vi "TargetExperimentalSetup_flux.vi"() -> ()   [LabVIEW 2015]
uses:
  <vilib>/userdefined/High Color/IMAQdx.ctl
  <vilib>/DAQmx/read.llb/DAQmx Read (Analog 1D DBL NChan 1Samp).vi
  <vilib>/DAQmx/read.llb/DAQmx Read (Analog DBL 1Chan 1Samp).vi
  <vilib>/DAQmx/miscellaneous.llb/DAQmx Fill In Error Info.vi
  <vilib>/Utility/file.llb/Write Delimited Spreadsheet (string).vi
  <instrlib>/Zaber A Series/Zaber A Series.lvlib
  <vilib>/vision/driver/NI_Vision_Acquisition_Software.lvlib
  <resource>/objmgr/imaqdx.rc
panel:
  in  "Y Coordinate":i32=50
  in  "X Coordinate":i32=50
  in  "Diameter":i32=10
  out "Image 2":T1(plugin-control)
  in  "Capture":bool
  out "Monochromatic Camera":errorcluster
  in  "Exposure Time (µs)":dbl=900000.0
  in  "Gamma Enabled":bool=TRUE
  in  "Frame Rate (hz)":dbl=24.0
  in  "Black Level":dbl(slide) scale=0.0..100.0
  out "Observer Camera":errorcluster
  in  "Exposure Time (µs)":dbl=100000.0
  in  "Gamma Enabled 2":bool=TRUE
  in  "Frame Rate (hz)":dbl=15.0
  in  "Black Level":dbl(slide) scale=0.0..100.0
  out "Flowmeter":errorcluster
  out "Thermocouple":errorcluster
  out "Actuator":errorcluster
  in  "Record":bool
  in  "Fluxmeter Data File":path
  in  "Image Folder Path":path
  out "Heat Flux (W/cm2)":string
  out "Fluxmeter":dbl(knob) scale=0.0..1200.0
  out "High Flux \nWarning":bool
  out "High Temp Warning":bool
  in  "Set Speed":bool
  out "Image":T1(plugin-control)
  in  "Step Increment (+/-)":string="10"
  out "Mass Flow (g/s)":string
  out "Mass Flow Inlet":dbl(knob) scale=0.0..150.0
  in  "Record Time (s)":u16=1 min=1
  in  "Lamp Number":dbl
  out "Filename":string
  in  "OK Button 2":bool
  out "Water Outlet - Fluxmeter":dbl(knob) scale=0.0..100.0
  out "Water Outlet - Target":dbl(knob) scale=0.0..100.0
  out "Water Inlet - Fluxmeter":dbl(knob) scale=0.0..100.0
  in  "?":bool
  out "High Temp Warning":bool
  out "High Temp \nWarning":bool
  out "Temperature (C°)":string
  out "Temperature (C°)":string
  out "Temperature (C°)":string
  out "End Reached":bool
  in  "?":bool
  out "Actuator Status":bool
  out "Position":string
  in  "?":bool
  in  "Speed (%)":string="35"
  in  "Set Position \n(150 <-> -150)":string="0"
  # "LINEAR ACTUATOR CONTROL"
  # "CAMERA FEEDS"
  # "CAMERA CONTROL"
  # "Monochromatic Camera"
  # "Observer Camera"
  # "HEAT FLUXMETER DISPLAY"
  # "HARDWARE CHECKLIST"
  # "NI 9211 THERMOCOUPLE MODULE DISPLAY"
  # "NI 9207 VOLTAGE AND CURRENT MODULE"
  # "Finding label on image"
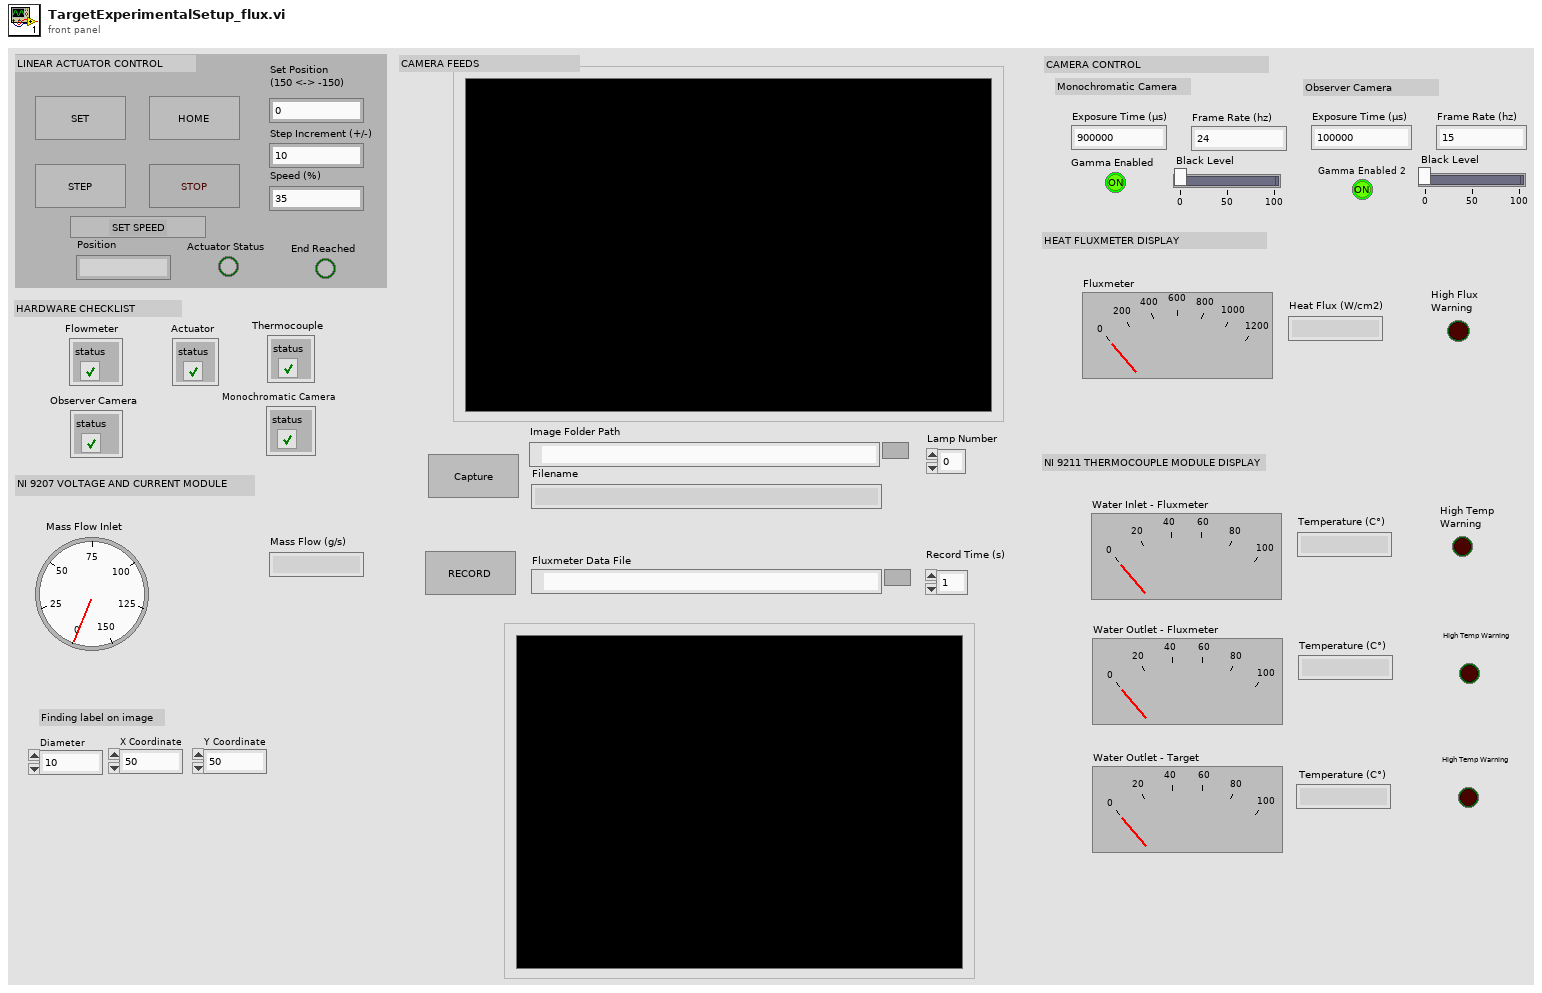
[diagram p1: front panel]
types:
  T1 = typedef "IMAQ Image.ctl" = refnum<image>
  T2 = cluster{"Left":i32, "Top":i32, "Right":i32, "Bottom":i32}
  T3 = typedef "IMAQdx.ctl" = refnum<k21>
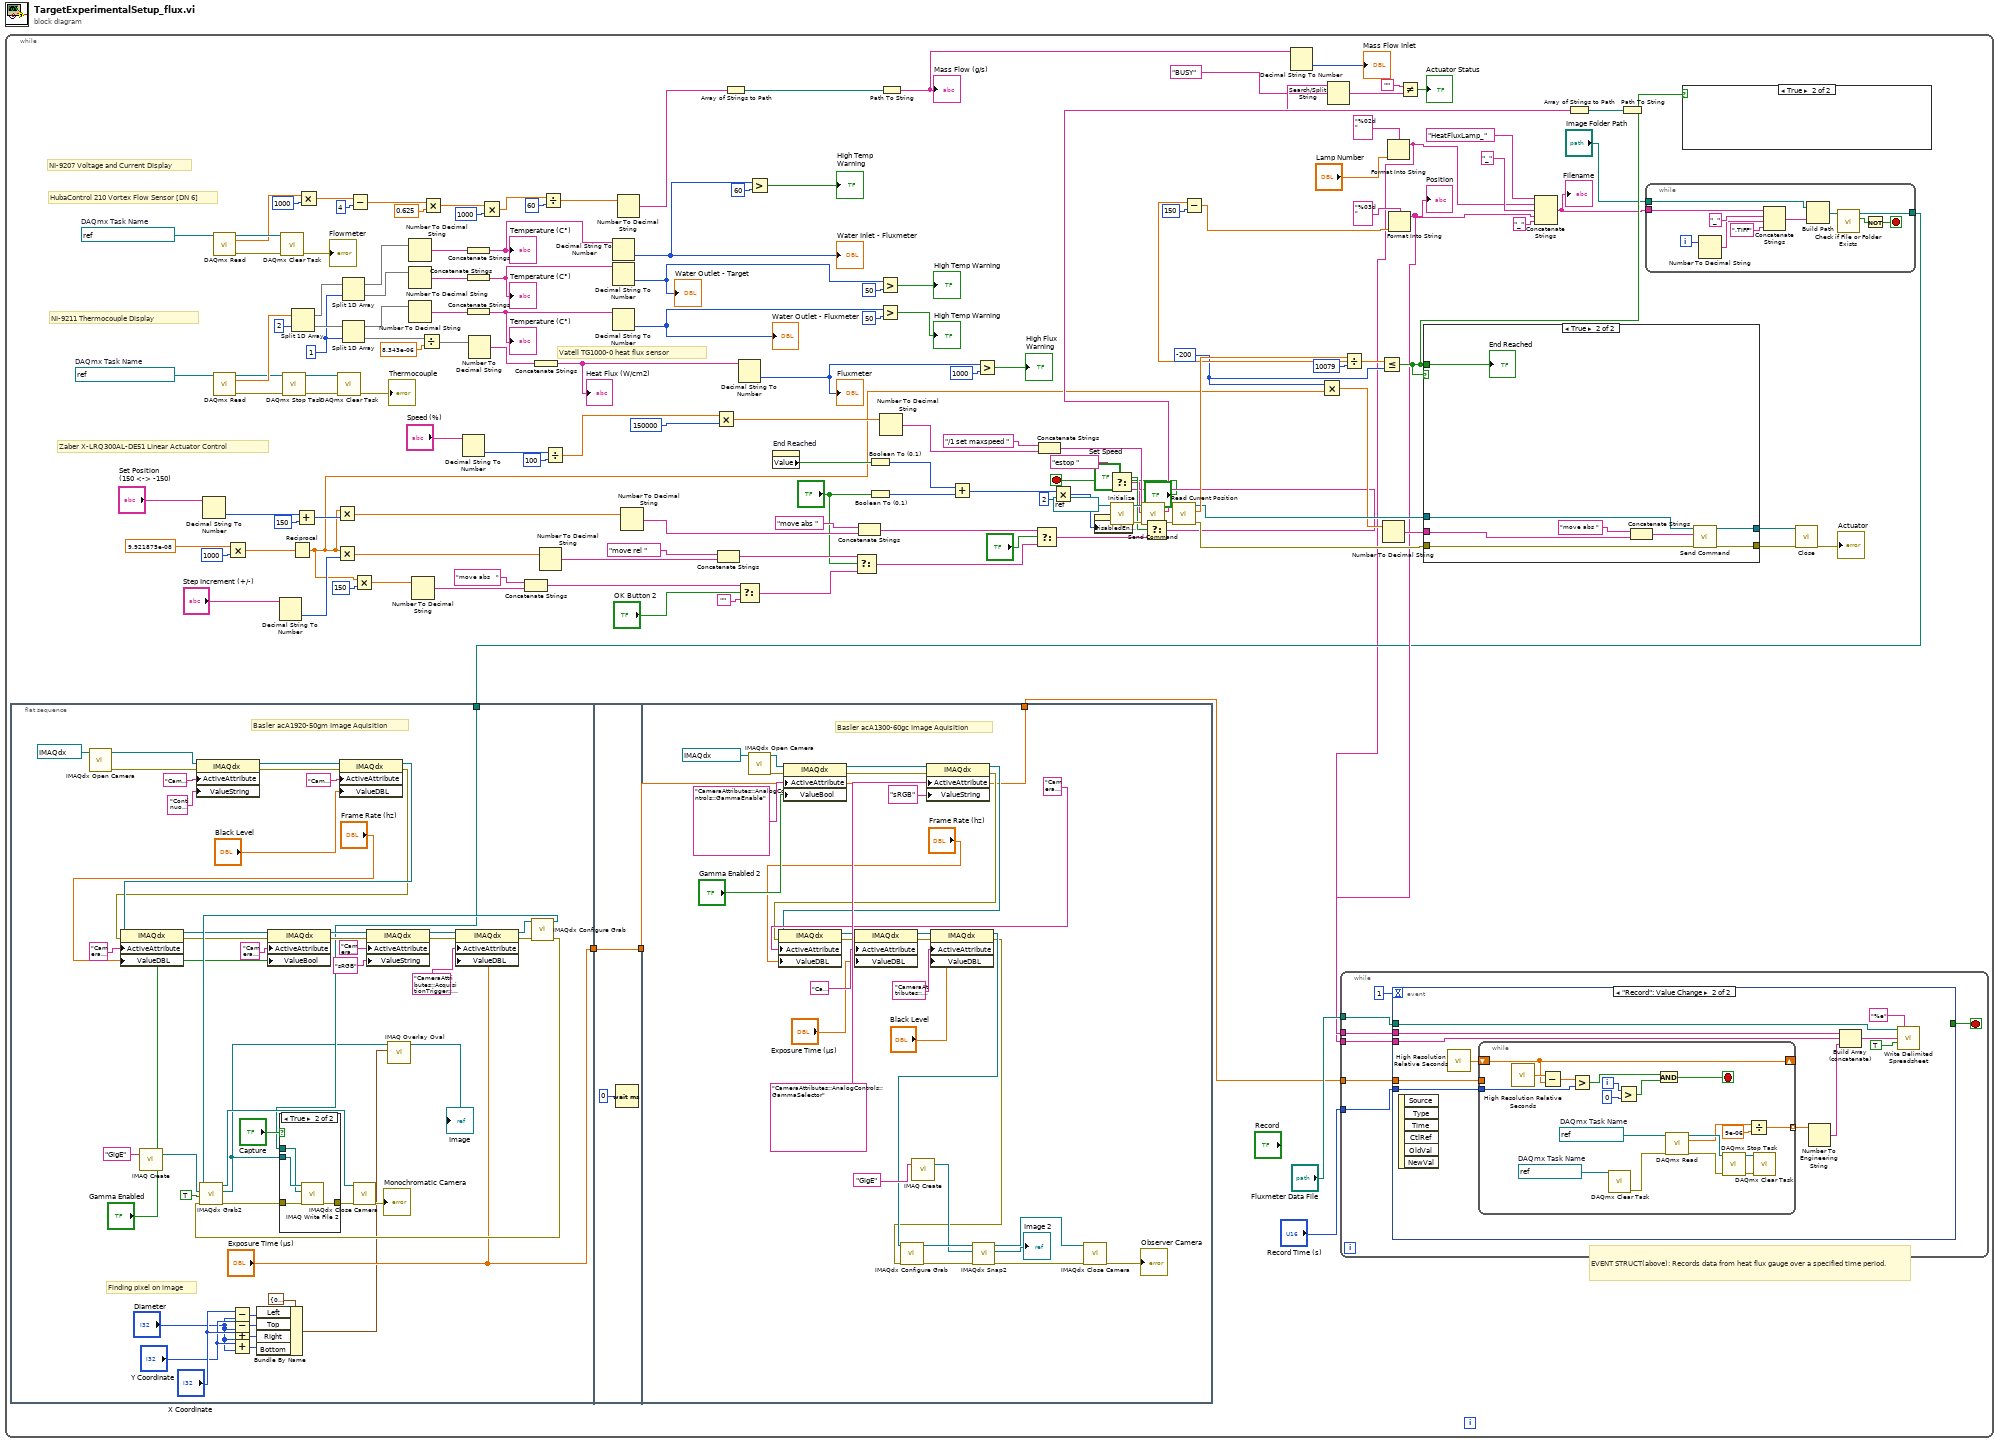
[diagram p0: block diagram]
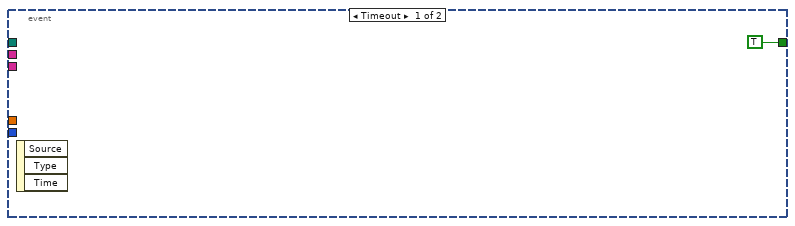
[diagram p3: hidden frame]
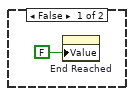
[diagram p4: hidden frame]
diagram:
  n1 = while {
    stop <- "?" stop-if-true
    w43 = refnum<k21> "Flowmeter-Current"  # DAQmx Task Name
    w103 = 1
    w35 = refnum<k21> "MyTemperatureTask"  # DAQmx Task Name
    w62 = -200
    # "Vatell TG1000-0 heat flux sensor"
    # "Zaber X-LRQ300AL-DE51 Linear Actuator Control"
    # "EVENT STRUCT(above): Records data from heat flux gauge over a specified time period."
    # "HubaControl 210 Vortex Flow Sensor [DN 6]"
    # "NI-9207 Voltage and Current Display"
    # "NI-9211 Thermocouple Display"
    n2 = flat-sequence {
      tunnel: ["Exposure Time (µs)"] -> w2
      tunnel: w4 -> [w161]
      tunnel: w2 -> [w202]
      tunnel: [w202] -> w1
      tunnel: [w204] -> w5
      tunnel: w1 -> [w204]
      frame #0 {
        # "Finding pixel on image"
        # "Basler acA1920-50gm Image Aquisition"
        n3 = call <vilib>:"IMAQdx Open Camera.vi"("Session In"=T3 "Mono" ("IMAQdx Session")) -> ("error out"=w169:errorcluster, "Session Out"=w170:T3)  [unwired: 9 in]
        n4 = call "IMAQ Create"("Image Name"="GigE") -> ("New Image"=w196:T1)  [unwired: 4 in, 1 out]
        n5 = property class="IMAQdx"(reference=w170, error in=w169, "ActiveAttribute"="CameraAttributes::AnalogControls::GainAuto", "ValueString"="Continuous") -> (reference out=w176:T3, error out=w174:errorcluster)
        n6 = Subtract(x="X Coordinate", y="Diameter") -> (x-y=w158:i32)
        n7 = Subtract(x="Y Coordinate", y="Diameter") -> (x-y=w155:i32)
        n8 = Add(x="X Coordinate", y="Diameter") -> (x+y=w156:i32)
        n9 = Add(x="Y Coordinate", y="Diameter") -> (x+y=w157:i32)
        n10 = Bundle By Name(cluster=T2 {"Left"=0, "Top"=0, "Right"=0, "Bottom"=0} ("Bounding Rectangle"), "Left"=w158, "Top"=w155, "Right"=w156, "Bottom"=w157) -> (w151:T2)
        n11 = property class="IMAQdx"(reference=w176, error in=w174, "ActiveAttribute"="CameraAttributes::AnalogControls::BlackLevelRaw", "ValueDBL"="Black Level") -> (reference out=w175:T3, error out=w173:errorcluster)
        n12 = property class="IMAQdx"(reference=w175, error in=w173, "ActiveAttribute"="CameraAttributes::AcquisitionTrigger::AcquisitionFrameRateAbs", "ValueDBL"="Frame Rate (hz)") -> (reference out=w179:T3, error out=w178:errorcluster)
        n13 = property class="IMAQdx"(reference=w179, error in=w178, "ActiveAttribute"="CameraAttributes::AnalogControls::GammaEnable", "ValueBool"="Gamma Enabled") -> (reference out=w191:T3, error out=w185:errorcluster)
        n14 = property class="IMAQdx"(reference=w191, error in=w185, "ActiveAttribute"="CameraAttributes::AnalogControls::GammaSelector", "ValueString"="sRGB") -> (reference out=w190:T3, error out=w184:errorcluster)
        n15 = property class="IMAQdx"(reference=w190, error in=w184, "ActiveAttribute"="CameraAttributes::AcquisitionTrigger::ExposureTimeAbs", "ValueDBL"="Exposure Time (µs)") -> (reference out=w188:T3, error out=w183:errorcluster)
        n16 = call <vilib>:"IMAQdx Configure Grab.vi"("error in"=w183, "Session In"=w188) -> ("error out"=w182:errorcluster, "Session Out"=w194:T3)  [unwired: 8 in]
        n17 = call <vilib>:"IMAQdx Grab2.vi"("error in"=w182, "Wait for Next Buffer? (Yes)"=TRUE, "Image In"=w196, "Session In"=w194) -> ("error out"=w163:errorcluster, "Image Out"=w150:T1, "Session Out"=w193:T3)  [unwired: 4 in, 1 out]
        n18 = case shown="True" "Capture" {
          tunnel: w150 -> [_ w199]
          tunnel: w163 -> [_ w201]
          tunnel: [_ w200] -> w162
          tunnel: w161 -> [_ w198]
          frame False {
          }
          frame True {
            n19 = call-poly "IMAQ Write File 2"("error in (no error)"=w201, "File Path"=w198, "Image"=w199) -> ("error out"=w200:errorcluster)  [unwired: 7 in, 1 out]
          }
        }
        n20 = call <vilib>:"IMAQdx Close Camera.vi"("error in"=w162, "Session In"=w193) -> ("error out"=→"Monochromatic Camera":errorcluster)  [unwired: 9 in]
        n21 = call "IMAQ Overlay Oval"("Bounding Rectangle"=w151, "Image"=w150) -> ("Image Out"=→"Image":T1)  [unwired: 8 in, 1 out]
      }
      frame #1 {
        n22 = Wait (ms)(milliseconds to wait=0) -> ()  [unwired: 1 out]
      }
      frame #2 {
        # "Basler acA1300-60gc Image Aquisition"
        n23 = call <vilib>:"IMAQdx Open Camera.vi"("Session In"=T3 "GIE1300-1" ("IMAQdx Session 2")) -> ("error out"=w215:errorcluster, "Session Out"=w216:T3)  [unwired: 9 in]
        n24 = property class="IMAQdx"(reference=w216, error in=w215, "ActiveAttribute"="CameraAttributes::AnalogControls::GammaEnable", "ValueBool"="Gamma Enabled 2") -> (reference out=w234:T3, error out=w231:errorcluster)
        n25 = call "IMAQ Create"("Image Name"="GigE") -> ("New Image"=w226:T1)  [unwired: 4 in, 1 out]
        n26 = property class="IMAQdx"(reference=w234, error in=w231, "ActiveAttribute"="CameraAttributes::AnalogControls::GammaSelector", "ValueString"="sRGB") -> (reference out=w221:T3, error out=w220:errorcluster)
        n27 = property class="IMAQdx"(reference=w221, error in=w220, "ActiveAttribute"="CameraAttributes::AcquisitionTrigger::AcquisitionFrameRateAbs", "ValueDBL"="Frame Rate (hz)") -> (reference out=w218:T3, error out=w217:errorcluster)
        n28 = property class="IMAQdx"(reference=w218, error in=w217, "ActiveAttribute"="CameraAttributes::AcquisitionTrigger::ExposureTimeAbs", "ValueDBL"="Exposure Time (µs)") -> (reference out=w212:T3, error out=w211:errorcluster)
        n29 = property class="IMAQdx"(reference=w212, error in=w211, "ActiveAttribute"="CameraAttributes::AnalogControls::BlackLevelRaw", "ValueDBL"="Black Level") -> (reference out=w208:T3, error out=w207:errorcluster)
        n30 = call <vilib>:"IMAQdx Configure Grab.vi"("error in"=w207, "Session In"=w208) -> ("error out"=w229:errorcluster, "Session Out"=w228:T3)  [unwired: 8 in]
        n31 = call <vilib>:"IMAQdx Snap2.vi"("error in"=w229, "Image In"=w226, "Session In"=w228) -> ("error out"=w223:errorcluster, "Image Out"=→"Image 2":T1, "Session Out"=w225:T3)  [unwired: 6 in]
        n32 = call <vilib>:"IMAQdx Close Camera.vi"("error in"=w223, "Session In"=w225) -> ("error out"=→"Observer Camera":errorcluster)  [unwired: 9 in]
      }
    }
    n33 = Decimal String To Number(string="Set Position \n(150 <-> -150)") -> (number=w91:i32)  [unwired: 2 in, 1 out]
    n34 = call-poly <vilib>:"DAQmx Read.vi"("task/channels in"=w43) -> ("task out"=w45:refnum<k21>, "data"=w34:dbl[], "error out"=w44:errorcluster)  [unwired: 12 in]
    n35 = call-poly <vilib>:"DAQmx Read.vi"("task/channels in"=w35) -> ("task out"=w16:refnum<k21>, "data"=w107:dbl[], "error out"=w15:errorcluster)  [unwired: 12 in]
    n36 = Multiply(x=9.921875e-08, y=1000) -> (x*y=w145:dbl)
    n37 = Decimal String To Number(string="Step Increment (+/-)") -> (number=w89:i32)  [unwired: 2 in, 1 out]
    n38 = call <vilib>:"DAQmx Clear Task.vi"("task in"=w45, "error in"=w44) -> ("error out"=→"Flowmeter":errorcluster)  [unwired: 13 in]
    n39 = call <vilib>:"DAQmx Stop Task.vi"("task/channels in"=w16, "error in"=w15) -> ("task out"=w14:refnum<k21>, "error out"=w13:errorcluster)  [unwired: 12 in]
    n40 = Reciprocal(x=w145) -> (1/x=w70:dbl)
    n41 = Split 1D Array(array=w107, index=2) -> (first subarray=w105:dbl[], second subarray=w104:dbl[])
    n42 = Add(x=w91, y=150) -> (x+y=w94:i32)
    n43 = Multiply(x=w34, y=1000) -> (x*y=w32:dbl[])
    n44 = Multiply(x=w70, y=w94) -> (x*y=w93:dbl)
    n45 = Multiply(x=w70, y=w89) -> (x*y=w130:dbl)
    n46 = call <vilib>:"DAQmx Clear Task.vi"("task in"=w14, "error in"=w13) -> ("error out"=→"Thermocouple":errorcluster)  [unwired: 13 in]
    n47 = Split 1D Array(array=w105, index=w103) -> (first subarray=w100:dbl[], second subarray=w102:dbl[])
    n48 = Split 1D Array(array=w104, index=w103) -> (first subarray=w101:dbl[], second subarray=w38:dbl[])
    n49 = Subtract(x=w32, y=4) -> (x-y=w48:dbl[])
    n50 = Multiply(x=w70, y=150) -> (x*y=w72:dbl)
    n51 = Number To Decimal String(number=w100) -> (decimal integer string=w26:string[])  [unwired: 1 in]
    n52 = Number To Decimal String(number=w102) -> (decimal integer string=w28:string[])  [unwired: 1 in]
    n53 = Number To Decimal String(number=w101) -> (decimal integer string=w30:string[])  [unwired: 1 in]
    n54 = Number To Decimal String(number=w72) -> (decimal integer string=w75:string)  [unwired: 1 in]
    n55 = Divide(x=w38, y=8.343e-06) -> (x/y=w17:dbl[])
    n56 = Multiply(x=w48, y=0.625) -> (x*y=w57:dbl[])
    n57 = Decimal String To Number(string="Speed (%)") -> (number=w82:i32)  [unwired: 2 in, 1 out]
    n58 = Concatenate Strings(w26) -> (w25:string)
    "Temperature (C°)" <- w25
    n59 = Concatenate Strings(w28) -> (w27:string)
    "Temperature (C°)" <- w27
    n60 = Concatenate Strings(w30) -> (w29:string)
    "Temperature (C°)" <- w29
    n61 = Number To Decimal String(number=w17) -> (decimal integer string=w31:string[])  [unwired: 1 in]
    n62 = Multiply(x=w57, y=1000) -> (x*y=w55:dbl[])
    n63 = Concatenate Strings("move abs   ", w75) -> (w71:string)
    n64 = Concatenate Strings(w31) -> (w7:string)
    "Heat Flux (W/cm2)" <- w7
    n65 = Number To Decimal String(number=w130) -> (decimal integer string=w128:string)  [unwired: 1 in]
    n66 = Divide(x=w55, y=60) -> (x/y=w58:dbl[])
    n67 = Divide(x=w82, y=100) -> (x/y=w79:dbl)
    n68 = Decimal String To Number(string=w25) -> (number=w61:i32)  [unwired: 2 in, 1 out]
    "Water Inlet - Fluxmeter" <- w61
    n69 = Decimal String To Number(string=w27) -> (number=w24:i32)  [unwired: 2 in, 1 out]
    "Water Outlet - Target" <- w24
    n70 = Decimal String To Number(string=w29) -> (number=w20:i32)  [unwired: 2 in, 1 out]
    "Water Outlet - Fluxmeter" <- w20
    n71 = Number To Decimal String(number=w58) -> (decimal integer string=w50:string[])  [unwired: 1 in]
    n72 = Number To Decimal String(number=w93) -> (decimal integer string=w143:string)  [unwired: 1 in]
    n73 = Multiply(x=w79, y=150000) -> (x*y=w78:dbl)
    n74 = Concatenate Strings("move rel ", w128) -> (w127:string)
    n75 = Array of Strings to Path(0:w50) -> (2:w51:path)  [unwired: 1 in]
    n76 = Decimal String To Number(string=w7) -> (number=w41:i32)  [unwired: 2 in, 1 out]
    "Fluxmeter" <- w41
    n77 = Select(t=w71, s="OK Button 2", f="") -> (s? t:f=w69:string)
    n78 = Greater?(x=w61, y=60) -> (0:→"High Temp \nWarning":bool)
    n79 = property on="End Reached" class="Bool (strict)"() -> ("Value"=w120:bool)  [unwired: 2 in, 2 out]
    n80 = Select(t=w127, s="?", f=w69) -> (s? t:f=w126:string)
    n81 = Concatenate Strings("move abs ", w143) -> (w125:string)
    n82 = Boolean To (0,1)(Boolean=w120) -> (0, 1=w119:i16)
    n83 = Boolean To (0,1)(Boolean="?") -> (0, 1=w121:i16)
    n84 = Greater?(x=w24, y=50) -> (0:→"High Temp Warning":bool)
    n85 = Greater?(x=w20, y=50) -> (0:→"High Temp Warning":bool)
    n86 = Number To Decimal String(number=w78) -> (decimal integer string=w86:string)  [unwired: 1 in]
    n87 = Path To String(path=w51) -> (string=w53:string)
    "Mass Flow (g/s)" <- w53
    n88 = Add(x=w119, y=w121) -> (x+y=w118:i16)
    n89 = Greater?(x=w41, y=1000) -> (0:→"High Flux \nWarning":bool)
    n90 = Select(t=w125, s="?", f=w126) -> (s? t:f=w83:string)
    n91 = Concatenate Strings("/1 set maxspeed ", w86) -> (w84:string)
    n92 = Multiply(x=w118, y=2) -> (x*y=w114:i32)
    n93 = property class="Bool"("DisabledEnum"=w114) -> ()  [unwired: 2 in, 2 out]
    n94 = call <instrlib>:"Initialize.vi"("VISA resource name"=refnum<visa-resource-name> "COM3") -> ("error out"=w113:errorcluster, "VISA resource name out"=w141:refnum<visa-resource-name>)  [unwired: 9 in]
    n95 = Select(t=w84, s="Set Speed", f=w83) -> (s? t:f=w67:string)
    n96 = Select(t="estop ", s="?", f=w67) -> (s? t:f=w66:string)
    n97 = call <instrlib>:"Send Command.vi"("error in (no error)"=w113, "Command"=w66, "VISA resource name"=w141) -> ("error out"=w112:errorcluster, "Response String Array"=w136:string[], "VISA resource name out"=w140:refnum<visa-resource-name>)  [unwired: 4 in, 2 out]
    n98 = call <instrlib>:"Read Current Position.vi"("error in (no error)"=w112, "VISA resource name"=w140) -> ("error out"=w111:errorcluster, "Position"=w139:dbl, "VISA resource name out"=w117:refnum<visa-resource-name>)  [unwired: 7 in]
    n99 = Decimal String To Number(string=w53) -> (number=→"Mass Flow Inlet":i32)  [unwired: 2 in, 1 out]
    n100 = Multiply(x=w62, y=w70) -> (x*y=w116:dbl)
    n101 = Divide(x=w139, y=10079) -> (x/y=w63:dbl)
    n102 = Subtract(x=w63, y=150) -> (x-y=w18:dbl)
    n103 = Less Or Equal?(x=w63, y=w62) -> (x <= y?=w64:bool)
    n104 = Number To Decimal String(number=w116) -> (decimal integer string=w115:string)  [unwired: 1 in]
    n105 = Format Into String(format string="%02d", "Lamp Number") -> (resulting string=w3:string)  [unwired: 2 in, 1 out]
    n106 = Format Into String(format string="%03d", w18) -> (resulting string=w9:string)  [unwired: 2 in, 1 out]
    "Position" <- w9
    n107 = while {
      tunnel: "Fluxmeter Data File" -> [w240]
      tunnel: w3 -> [w239]
      tunnel: w9 -> [w238]
      tunnel: w5 -> [w237]
      tunnel: "Record Time (s)" -> [w236]
      stop <- w241 stop-if-true
      n108 = event shown="[1] \"Record\": Value Change" {
        selector: _ -> [_ _]
        dyn-events: _ -> [_ _]
        timeout: 1 -> [_ _]
        tunnel: [TRUE _] -> w241
        tunnel: w240 -> [_ w254]
        tunnel: w239 -> [_ w250]
        tunnel: w238 -> [_ w249]
        tunnel: w237 -> [_ w247]
        tunnel: w236 -> [_ w244]
        event Timeout {
          n109 = event-data() -> ()  [unwired: 1 in, 3 out]
        }
        event "Record": Value Change {
          n110 = event-data() -> ()  [unwired: 1 in, 6 out]
          n111 = call <vilib>:"High Resolution Relative Seconds.vi"() -> ("relative seconds"=w246:dbl)
          n112 = while {
            tunnel: [w257] -> w252 mode=indexing
            shift-right: [w259] -> _
            shift-left: w246 -> [w259]
            tunnel: w247 -> [_]
            tunnel: w244 -> [w255]
            i -> [w266]
            stop <- w261 stop-if-true
            w268 = refnum<k21> "HF-Voltage"  # DAQmx Task Name
            w273 = refnum<k21> "HF-Voltage"  # DAQmx Task Name
            n113 = call <vilib>:"High Resolution Relative Seconds.vi"() -> ("relative seconds"=w260:dbl)
            n114 = Subtract(x=w260, y=w259) -> (x-y=w264:dbl)
            n115 = Greater?(x=w264, y=w255) -> (0:w263:bool)
            n116 = call <vilib>:"DAQmx Clear Task.vi"("task in"=w268) -> ("error out"=w267:errorcluster)  [unwired: 14 in]
            n117 = Greater?(x=w266, y=0) -> (0:w262:bool)
            n118 = And(x=w263, y=w262) -> (x .and. y?=w261:bool)
            n119 = call-poly <vilib>:"DAQmx Read.vi"("task/channels in"=w273, "error in"=w267) -> ("task out"=w272:refnum<k21>, "data"=w256:dbl, "error out"=w271:errorcluster)  [unwired: 11 in]
            n120 = call <vilib>:"DAQmx Stop Task.vi"("task/channels in"=w272, "error in"=w271) -> ("task out"=w270:refnum<k21>, "error out"=w269:errorcluster)  [unwired: 12 in]
            n121 = Divide(x=w256, y=9e-06) -> (x/y=w257:dbl)
            n122 = call <vilib>:"DAQmx Clear Task.vi"("task in"=w270, "error in"=w269) -> ()  [unwired: 13 in, 1 out]
          }
          n123 = Number To Engineering String(4:w252) -> (0:w251:string[])  [unwired: 3 in]
          n124 = Build Array (concatenate)(w249, w250, w251) -> (w248:string[])
          n125 = call-poly <vilib>:"Write Delimited Spreadsheet.vi"("file path (dialog if empty)"=w254, "format (%s)"="%e", "1D data"=w248, "append to file? (F)"=TRUE) -> ()  [unwired: 10 in, 2 out]
        }
      }
    }
    n126 = case shown="True" w64 {
      tunnel: w64 -> [_ w293]
      tunnel: w117 -> [_ w292]
      tunnel: w115 -> [_ w289]
      tunnel: w111 -> [_ w288]
      tunnel: [_ w287] -> w110
      tunnel: [_ w286] -> w108
      frame False {
      }
      frame True {
        n127 = Concatenate Strings("move abs ", w289) -> (w290:string)
        n128 = call <instrlib>:"Send Command.vi"("error in (no error)"=w288, "Command"=w290, "VISA resource name"=w292) -> ("error out"=w287:errorcluster, "VISA resource name out"=w286:refnum<visa-resource-name>)  [unwired: 4 in, 3 out]
        "End Reached" <- w293
      }
    }
    n129 = Concatenate Strings("HeatFluxLamp_", w3, "_", w9, "_") -> (w36:string)
    "Filename" <- w36
    n130 = Array of Strings to Path(0:w136) -> (2:w137:path)  [unwired: 1 in]
    n131 = Path To String(path=w137) -> (string=w135:string)
    n132 = Search/Split String(string=w135, search string/char (-)="BUSY") -> (match + rest of string=w133:string)  [unwired: 1 in, 2 out]
    n133 = Not Equal?(x="", y=w133) -> (x != y?=→"Actuator Status":bool)
    n134 = while {
      tunnel: "Image Folder Path" -> [w280]
      tunnel: [w279] -> w4
      tunnel: w36 -> [w278]
      i -> [w275]
      stop <- w282 stop-if-true
      n135 = Number To Decimal String(number=w275) -> (decimal integer string=w274:string)  [unwired: 1 in]
      n136 = Concatenate Strings(w278, "_", w274, ".TIFF") -> (w284:string)
      n137 = Build Path(base path=w280, name or relative path=w284) -> (appended path=w283:path)
      n138 = call <vilib>:"Check if File or Folder Exists.vi"("path"=w283) -> ("file or folder exists?"=w281:bool, "dup path"=w279:path)  [unwired: 8 in, 1 out]
      n139 = Not(x=w281) -> (.not. x?=w282:bool)
    }
    n140 = case shown="True" w64 {
      frame False {
        n141 = property on="End Reached" class="Bool (strict)"("Value"=FALSE) -> ()  [unwired: 2 in, 2 out]
      }
      frame True {
      }
    }
    n142 = call <instrlib>:"Close.vi"("error in (no error)"=w110, "VISA resource name"=w108) -> ("error out"=→"Actuator":errorcluster)  [unwired: 9 in]
  }
